vi "CamTestGetEvntsResponse.vi"(8 "error in (no error)":errorcluster, 10 "CameraTestingEvnt":T1, 11 "ICameraTestingUI in":refnum<class "ICameraTestingUI.lvclass">) -> (0 "error out":errorcluster, 3 "ICameraTestingUI out":refnum<class "ICameraTestingUI.lvclass">)   [LabVIEW 2020, in "ICameraTestingUI.lvlib" / "ICameraTestingUI.lvclass"]
uses:
  ICameraTestingUI.lvclass
  ICameraTesting/TypeDef/Events.ctl
  Camera/ICamera/TypeDef/SnapInfo.ctl
  ICameraTesting/TypeDef/FrameRateValReceived.ctl
  ICameraTesting/TypeDef/ImgTypeValReceived.ctl
  ICameraTesting/TypeDef/ResolutionValReceived.ctl
  ICameraTesting/TypeDef/VideoOptCodesUpdated.ctl
  ICameraTesting/TypeDef/VideoOptionsInfo.ctl
  ICameraTesting/TypeDef/StatusUpdated.ctl
  ICameraTesting/TypeDef/StatusRecord.ctl
  ICameraTesting/TypeDef/VideoBufferUpdate.ctl
  Camera/ICamera/TypeDef/ICamera_typedef.lvlib
  ICameraTesting/TypeDef/ICameraTesting_typedef.lvlib
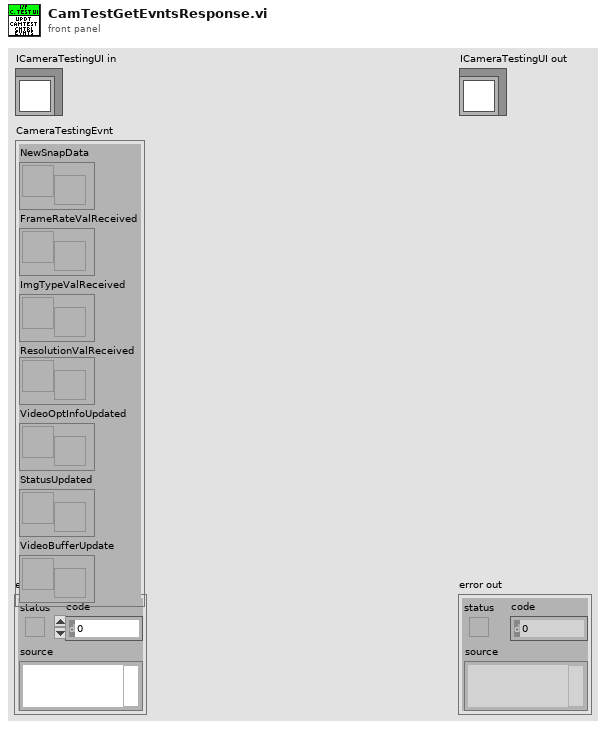
[diagram p1: front panel]
types:
  T1 = typedef "ICameraTesting_typedef.lvlib/Events.ctl" = cluster{"NewSnapData":refnum<user-event>, "FrameRateValReceived":T2, "ImgTypeValReceived":T3, "ResolutionValReceived":T4, "VideoOptInfoUpdated":T5, "StatusUpdated":T6, "VideoBufferUpdate":T7}
  T2 = typedef "ICameraTesting_typedef.lvlib/FrameRateValReceived.ctl" = refnum<user-event>
  T3 = typedef "ICameraTesting_typedef.lvlib/ImgTypeValReceived.ctl" = refnum<user-event>
  T4 = typedef "ICameraTesting_typedef.lvlib/ResolutionValReceived.ctl" = refnum<user-event>
  T5 = typedef "ICameraTesting_typedef.lvlib/VideoOptCodesUpdated.ctl" = refnum<user-event>
  T6 = typedef "ICameraTesting_typedef.lvlib/StatusUpdated.ctl" = refnum<user-event>
  T7 = typedef "ICameraTesting_typedef.lvlib/VideoBufferUpdate.ctl" = refnum<user-event>
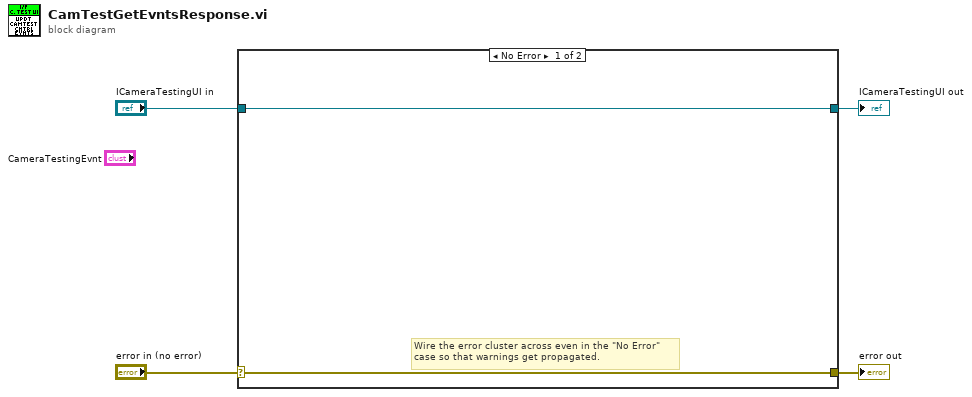
[diagram p0: block diagram]
diagram:
  n1 = case shown="No Error" "error in (no error)" {
    selector: "error in (no error)" -> [w5 w8]
    tunnel: [w5 w8] -> w3
    tunnel: [w6 w7] -> w1
    tunnel: "ICameraTestingUI in" -> [w6 w7]
    frame No Error {
      # "Wire the error cluster across even in the \"No Error\"\ncase so that warnings get propagated."
    }
    frame Error {
    }
  }
  "error out" <- w3
  "ICameraTestingUI out" <- w1
